vi "Panel.vi"(11 "AppDetailPanel in":refnum<class "AppDetailPanel.lvclass">) -> ()   [LabVIEW 2020, in "PicoG-App.lvlib" / "AppDetailPanel.lvclass"]
uses:
  AppDetailPanel.lvclass
  C:/Program Files (x86)/National Instruments/LabVIEW 2020/vi.lib/IlluminatedG/IG OOPanel/OOPanel/Panel/Panel.lvclass
  <vilib>/IlluminatedG/IG OOPanel/OOPanel/Panel/Basic UI State.ctl
  AppDetailPanel.lvclass/AppDetailPanel.ctl
  <vilib>/IlluminatedG/IG OOPanel/OOPanel/Panel/Panel.lvclass
  <vilib>/IlluminatedG/IG OOPanel/OOPanel/OOPanel.lvlib
  ViaApp/ViaApp.lvclass
panel:
  in  "Deploy":bool
  in  "Device":string(combo)="<No Configured Devices>"
  out "Name":string
  in  "Explore":bool
  out "App Path":path
  out "Source":string
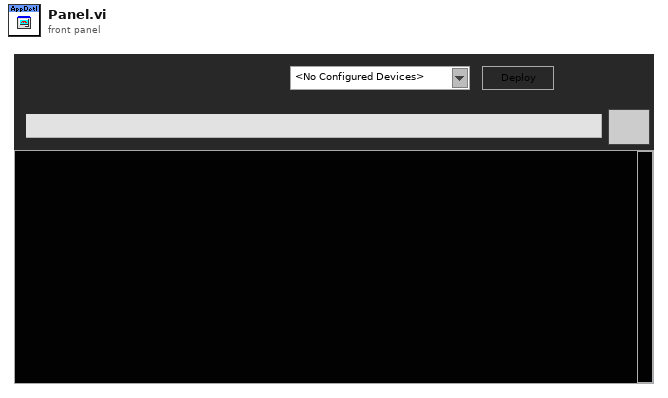
[diagram p1: front panel]
types:
  T1 = typedef "OOPanel.lvlib/Panel.lvclass/Basic UI State.ctl" = enum16{"Init", "Run", "Close"}
  T2 = typedef "PicoG-App.lvlib/AppDetailPanel.lvclass/Incoming Events.ctl" = cluster{"App Updated":refnum<user-event>}
  T3 = typedef "OOPanel.lvlib/Panel.lvclass/Panel Events.ctl" = cluster{"Visbility":refnum<user-event>, "Close":refnum<user-event>}
  T4 = typedef "PicoG-App.lvlib/AppDetailPanel.lvclass/Ref Data.ctl" = cluster{"App":refnum<class "ViaApp.lvclass">}
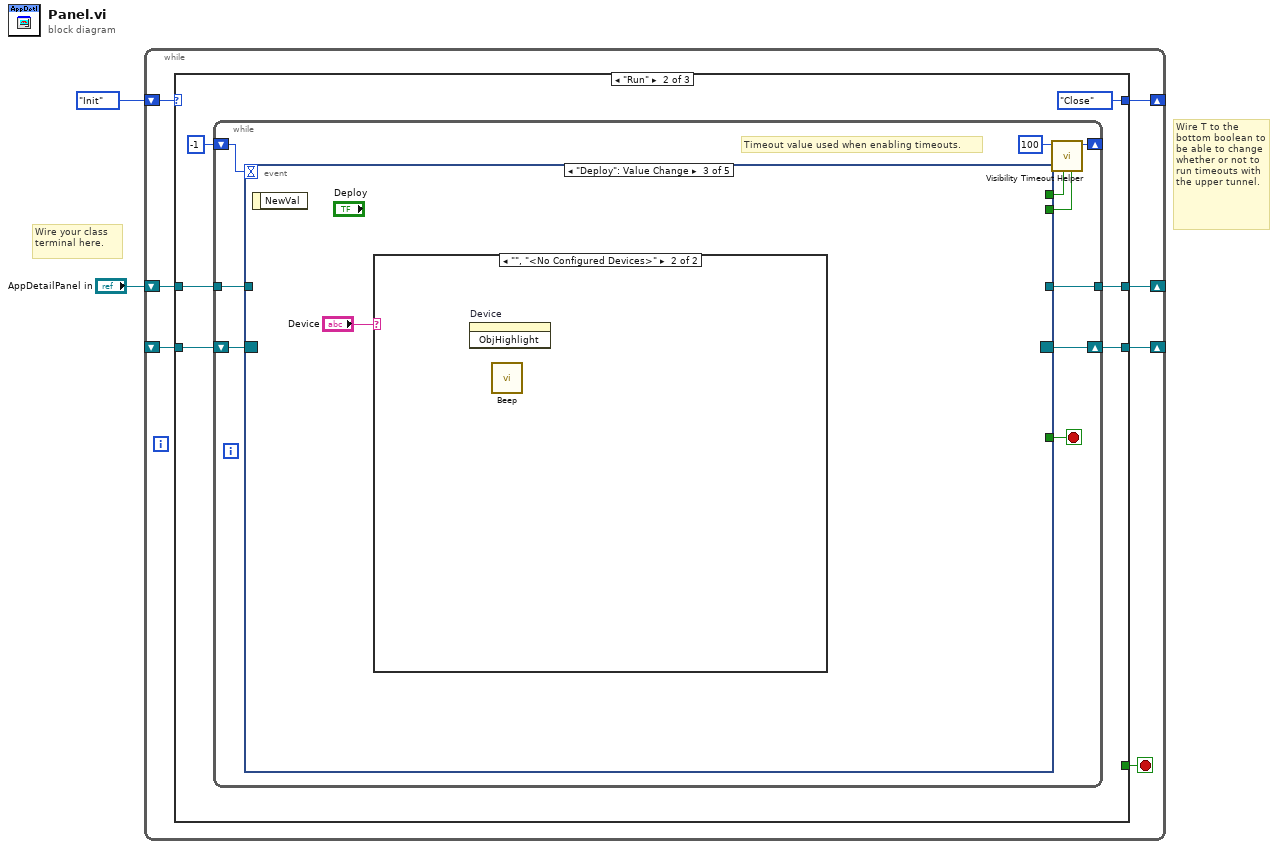
[diagram p0: block diagram]
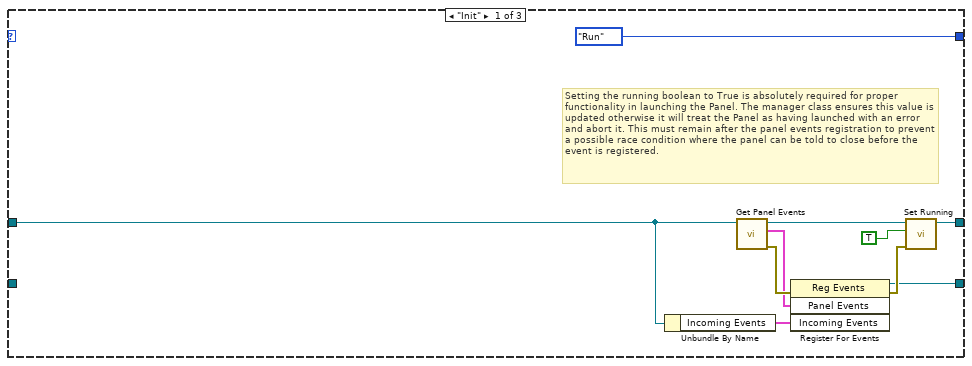
[diagram p2: hidden frame]
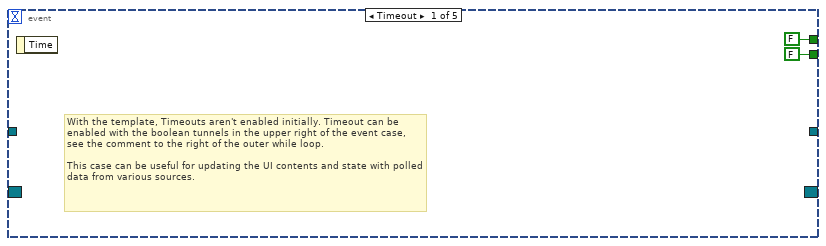
[diagram p3: hidden frame]
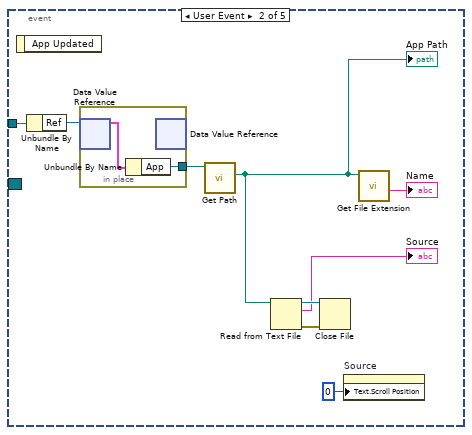
[diagram p4: hidden frame]
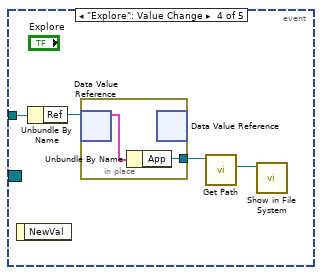
[diagram p6: hidden frame]
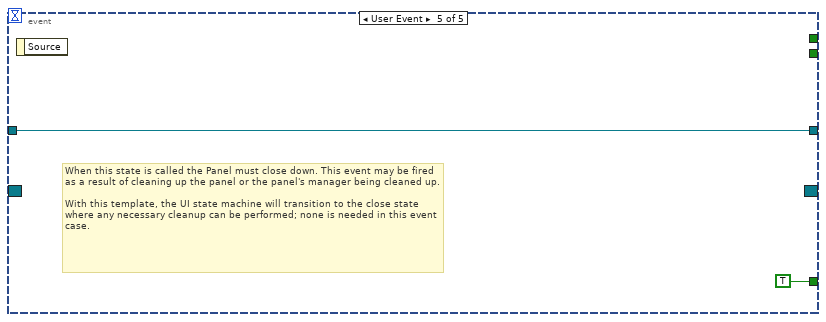
[diagram p7: hidden frame]
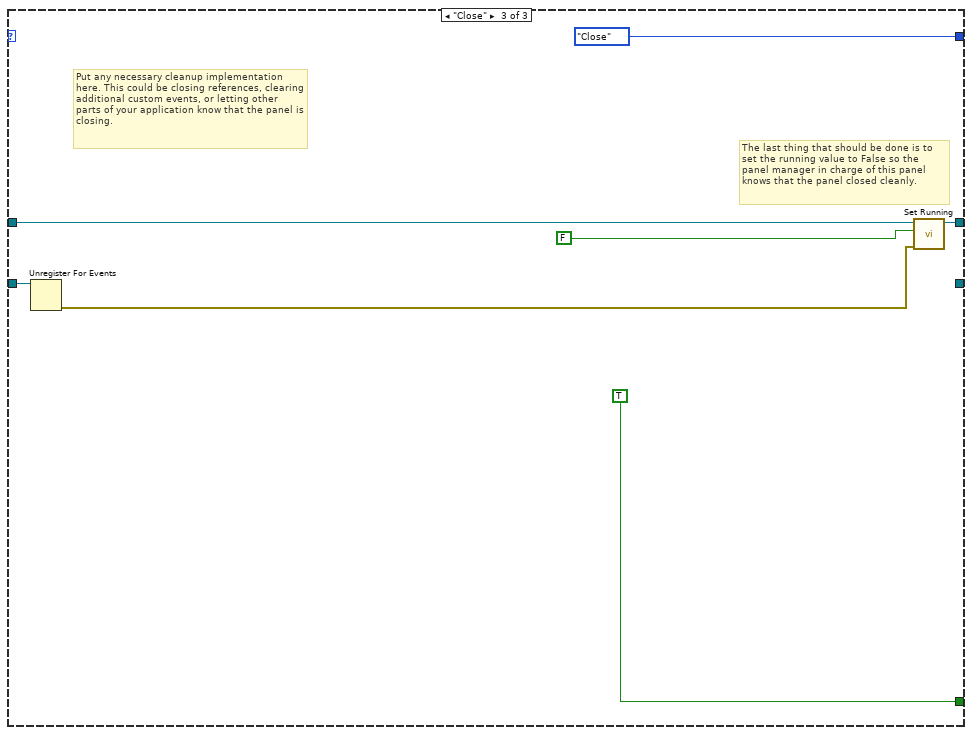
[diagram p8: hidden frame]
diagram:
  # "Wire T to the bottom boolean to be able to change whether or not to run timeouts with the upper tunnel."
  # "Wire your class terminal here."
  n1 = while {
    shift-right: [w8] -> _
    shift-left: _ -> [w9]
    shift-right: [w6] -> _
    shift-left: Basic_UI_State."Init" ("Basic UI State") -> [w7]
    shift-right: [w4] -> _
    shift-left: "AppDetailPanel in" -> [w3]
    stop <- w5 stop-if-true
    n2 = case shown="\"Run\"" w7 {
      tunnel: w9 -> [_ w25 w60]
      tunnel: [w13 w23 _] -> w8
      tunnel: [Basic_UI_State."Run" ("Basic UI State") Basic_UI_State."Close" ("Basic UI State") Basic_UI_State."Close" ("Basic UI State")] -> w6
      tunnel: [_ _ TRUE] -> w5
      tunnel: [w12 w20 w58] -> w4
      tunnel: w3 -> [w11 w21 w59]
      frame "Init" {
        # "Setting the running boolean to True is absolutely required for proper functionality in launching the Panel. The manager class ensures this value is updated otherwise it will treat the Panel as having launched with an error and abort it. This must remain after the panel events registration to prevent a possible race condition where the panel can be told to close before the event is registered."
        n3 = Unbundle By Name(w11) -> ("Incoming Events"=w10:T2)
        n4 = call <vilib>:"Get Panel Events.vi"("Panel in"=w11) -> ("error out"=w19:errorcluster, "Panel Events"=w15:T3, "Panel out"=w16:refnum<class "AppDetailPanel.lvclass">)  [unwired: 8 in]
        n5 = register-events(error in=w19, w15, w10) -> (reference out=w13:refnum<event-registration>, error out=w17:errorcluster)  [unwired: 1 in]
        n6 = call <vilib>:"Set Running.vi"("error in (no error)"=w17, "Running"=TRUE, "Panel in"=w16) -> ("Panel out"=w12:refnum<class "AppDetailPanel.lvclass">)  [unwired: 7 in, 1 out]
      }
      frame "Run" {
        n7 = while {
          shift-right: [w31] -> w23
          shift-left: w25 -> [w32]
          shift-right: [w34] -> _
          shift-left: -1 ("Timeout") -> [w33]
          tunnel: w21 -> [w27]
          tunnel: [w26] -> w20
          stop <- w28 stop-if-true
          # "Timeout value used when enabling timeouts."
          n8 = event shown="[2] \"Deploy\": Value Change" {
            selector: w32 -> [_ _ _ _ _]
            dyn-events: [_ _ _ _ _] -> w31
            timeout: w33 -> [_ _ _ _ _]
            tunnel: [FALSE _ _ _ _] -> w30
            tunnel: [FALSE _ _ _ _] -> w29
            tunnel: [_ _ _ _ TRUE] -> w28
            tunnel: w27 -> [_ w45 _ w51 w56]
            tunnel: [_ _ _ _ w56] -> w26
            event Timeout {
              # "With the template, Timeouts aren't enabled initially. Timeout can be enabled with the boolean tunnels in the upper right of the event case, see the comment to the right of the outer while loop.\n\nThis case can be useful for updating the UI contents and state with polled data from various sources."
              n9 = event-data() -> ()  [unwired: 1 in, 1 out]
            }
            event User Event {
              n10 = event-data() -> ()  [unwired: 1 in, 1 out]
              n11 = Unbundle By Name(w45) -> ("Ref"=w46:refnum<data-value>)
              n12 = in-place {
                in-place-border: [w47] -> w44
                n13 = in-place-dvr #1(w46) -> (w48:T4)  [unwired: 1 out]
                n14 = Unbundle By Name(w48) -> ("App"=w47:refnum<class "ViaApp.lvclass">)
                n15 = in-place-dvr #1() -> ()  [unwired: 1 in, 2 out]
              }
              n16 = call "Get Path.vi"("ViaApp in"=w44) -> ("Path"=w42:path)  [unwired: 8 in, 2 out]
              "App Path" <- w42
              n17 = Read from Text File(file (use dialog)=w42) -> (refnum out=w41:refnum<file>, text=→"Source":string, error out=w40:errorcluster)  [unwired: 3 in, 1 out]
              n18 = Close File(refnum=w41, error in=w40) -> ()  [unwired: 2 out]
              n19 = property on="Source" class="Str"("Text.Scroll Position"=u32 0) -> ()  [unwired: 2 in, 2 out]
              n20 = call <vilib>:"Get File Extension.vi"("file"=w42) -> ("filename without extension"=→"Name":string)  [unwired: 6 in, 4 out]
            }
            event "Deploy": Value Change {
              n21 = event-data() -> ()  [unwired: 1 in, 1 out]
              n22 = case shown="\"\", \"<No Configured Devices>\"" "Device" {
                frame Default {
                }
                frame "", "<No Configured Devices>" {
                  n23 = invoke on="Device" class="CmbBox" method="ObjHighlight"() -> ()  [unwired: 3 in, 3 out]
                  n24 = call <vilib>:"Beep.vi"() -> ()  [unwired: 12 in]
                }
              }
            }
            event "Explore": Value Change {
              n25 = event-data() -> ()  [unwired: 1 in, 1 out]
              n26 = Unbundle By Name(w51) -> ("Ref"=w53:refnum<data-value>)
              n27 = in-place {
                in-place-border: [w54] -> w52
                n28 = in-place-dvr #2(w53) -> (w55:T4)  [unwired: 1 out]
                n29 = Unbundle By Name(w55) -> ("App"=w54:refnum<class "ViaApp.lvclass">)
                n30 = in-place-dvr #2() -> ()  [unwired: 1 in, 2 out]
              }
              n31 = call "Get Path.vi"("ViaApp in"=w52) -> ("Path"=w50:path)  [unwired: 8 in, 2 out]
              n32 = call <vilib>:"Show in File System.vi"("file or directory path"=w50) -> ()  [unwired: 10 in, 1 out]
            }
            event User Event {
              # "When this state is called the Panel must close down. This event may be fired as a result of cleaning up the panel or the panel's manager being cleaned up.\n\nWith this template, the UI state machine will transition to the close state where any necessary cleanup can be performed; none is needed in this event case."
              n33 = event-data() -> ()  [unwired: 1 in, 1 out]
            }
          }
          n34 = call <vilib>:"Visibility Timeout Helper.vi"("Update?"=w29, "Use Timeout?"=w30, "Visible Timeout mS"=100) -> ("Timeout"=w34:i32)  [unwired: 8 in]
        }
      }
      frame "Close" {
        # "Put any necessary cleanup implementation here. This could be closing references, clearing additional custom events, or letting other parts of your application know that the panel is closing."
        # "The last thing that should be done is to set the running value to False so the panel manager in charge of this panel knows that the panel closed cleanly."
        n35 = Unregister For Events(event registration refnum=w60) -> (error out=w62:errorcluster)  [unwired: 1 in]
        n36 = call <vilib>:"Set Running.vi"("error in (no error)"=w62, "Running"=FALSE, "Panel in"=w59) -> ("Panel out"=w58:refnum<class "AppDetailPanel.lvclass">)  [unwired: 7 in, 1 out]
      }
    }
  }
